vi "Digital Write Square Wave.vi"(7 "Duration (ms)":u32, 8 "Error In":errorcluster, 9 "Frequency":u32, 10 "DO Channel":u8, 11 "LINX Device Config":T1) -> (0 "Error Out":errorcluster, 3 "LINX Device Config":T1)   [LabVIEW 2020, in "Device.lvlib"]
uses:
  Device.lvlib
  Type Defs/Error Type.ctl
  LMH-LINX.lvlib
  Type Defs/Interface.ctl
  Type Defs/Channels.ctl
  Type Defs/TCP Config.ctl
  Type Defs/LINX Device Config.ctl
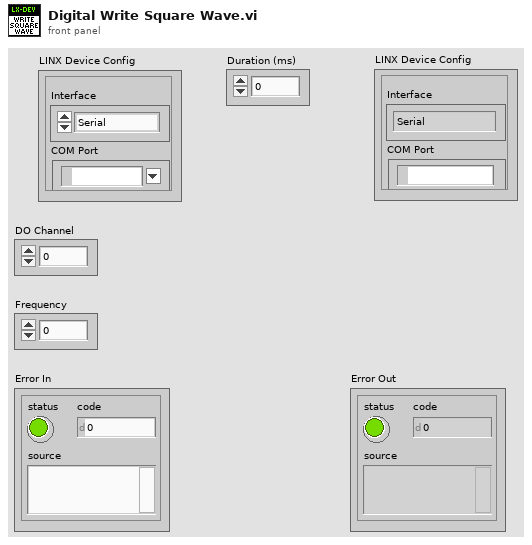
[diagram p1: front panel]
types:
  T1 = typedef "Device.lvlib/LINX Device Config.ctl" = cluster{"Interface":T2, "COM Port":refnum<visa-resource-name>, "TCP Configuration":T3, "Device Family":u8, "Device ID":u8, "Device Name":string, "TCP Ref":refnum<k5>, "Channels":T4}
  T2 = typedef "LMH-LINX.lvlib/Interface.ctl" = enum16{"Serial", "TCP"}
  T3 = typedef "Device.lvlib/TCP Config.ctl" = cluster{"IP Address":string, "Port":u16}
  T4 = typedef "LMH-LINX.lvlib/Channels.ctl" = cluster{"DI":u8[], "DO":u8[], "AI":u8[], "AO":u8[], "PWM":u8[], "QE":u8[], "UART":u8[], "I2C 2":u8[], "SPI":u8[], "CAN":u8[], "Servo":u8[], "AI Ref (V)":dbl, "AI Resolution (Bits)":u8, "AO Ref (V)":dbl, "AO Resolution (Bits)":u8}
  T5 = typedef "LMH-LINX.lvlib/Error Type.ctl" = enum16{"Unknown", "Timeout", "Corrupt Return Packet", "Unable To Connect", "Command Not Supported", "Channel DNE", "Invalid COM Config", "Firmware Version Mismatch", "myRIO Support", "CMD Specific Error", "Local IO Not Supported"}
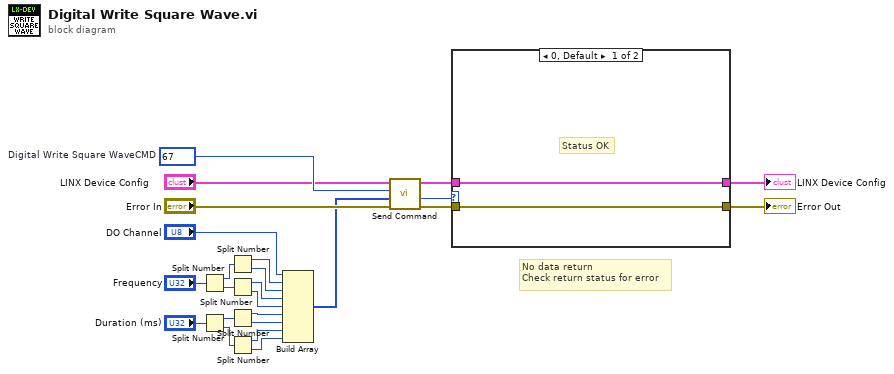
[diagram p0: block diagram]
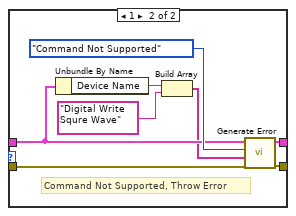
[diagram p2: hidden frame]
diagram:
  w23 = u16 67  # Digital Write Square WaveCMD
  # "No data return\nCheck return status for error"
  n1 = Split Number(x="Frequency") -> (hi(x)=w11:u16, lo(x)=w10:u16)
  n2 = Split Number(x="Duration (ms)") -> (hi(x)=w12:u16, lo(x)=w13:u16)
  n3 = Split Number(x=w11) -> (hi(x)=w8:u8, lo(x)=w7:u8)
  n4 = Split Number(x=w10) -> (hi(x)=w6:u8, lo(x)=w5:u8)
  n5 = Split Number(x=w12) -> (hi(x)=w4:u8, lo(x)=w3:u8)
  n6 = Split Number(x=w13) -> (hi(x)=w2:u8, lo(x)=w1:u8)
  n7 = Build Array("DO Channel", w8, w7, w6, w5, w4, w3, w2, w1) -> (w15:u8[])
  n8 = call "Send Command.vi"("Error In"="Error In", "ARGS"=w15, "CMD"=w23, "LINX Device Config"="LINX Device Config") -> ("Error Out"=w20:errorcluster, "Status"=w17:u8, "LINX Device Config"=w18:T1)  [unwired: 4 in, 1 out]
  n9 = case shown="0, Default" w17 {
    tunnel: [w26 w32] -> w22
    tunnel: w18 -> [w26 w28]
    tunnel: [w25 w33] -> w21
    tunnel: w20 -> [w25 w34]
    frame 0, Default {
      # "Status OK"
    }
    frame 1 {
      # "Command Not Supported, Throw Error"
      n10 = Unbundle By Name(w28) -> ("Device Name"=w30:string)
      n11 = Build Array(w30, "Digital Write Squre Wave") -> (w27:string[])
      n12 = call "Generate Error.vi"("Error In"=w34, "Arguments"=w27, "Error Type"=Error_Type."Command Not Supported", "LINX Device Config"=w28) -> ("Error Out"=w33:errorcluster, "Dup LINX Device Config"=w32:T1)  [unwired: 6 in]
    }
  }
  "Error Out" <- w21
  "LINX Device Config" <- w22
